vi "Quit With Parameter Code.vi"   [LabVIEW 2024, in "Integration Tests.lvlib"]
uses:
  Integration Tests.lvlib
  CLI Class/CLI.lvclass
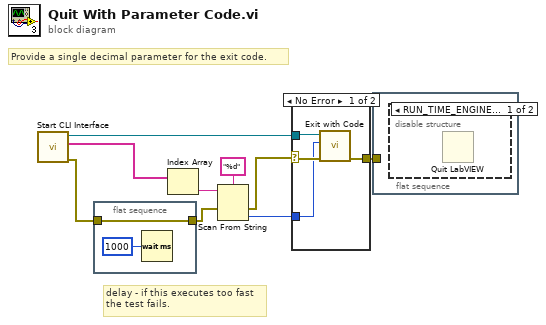
[diagram p0: block diagram]
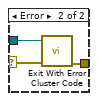
[diagram p2: hidden frame]
diagram:
  # "delay - if this executes too fast\nthe test fails."
  # "Provide a single decimal parameter for the exit code."
  n1 = call "Start CLI Interface.vi"() -> ("error out"=w2:errorcluster, "Custom Parameters"=w7:string[], "CLI out"=w9:refnum<class "CLI.lvclass">)  [unwired: 8 in, 1 out]
  n2 = flat-sequence {
    tunnel: w2 -> [w10]
    tunnel: [w10] -> w1
    frame #0 {
      n3 = Wait (ms)(milliseconds to wait=u32 1000) -> ()  [unwired: 1 out]
    }
  }
  n4 = Index Array(array=w7) -> (element=w6:string)  [unwired: 1 in]
  n5 = Scan From String(format string="%d", input string=w6, error in=w1) -> (error out=w4:errorcluster, output 1=w3:i32)  [unwired: 2 in, 2 out]
  n6 = case shown="No Error" w4 {
    selector: w4 -> [w14 w16]
    tunnel: w9 -> [w13 w18]
    tunnel: [w15 w17] -> w8
    tunnel: w3 -> [w12 _]
    frame No Error {
      n7 = call "Exit with Code.vi"("error in (no error)"=w14, "Exit Code (0)"=w12, "CLI in"=w13) -> ("error out"=w15:errorcluster)  [unwired: 8 in]
    }
    frame Error {
      n8 = call "Exit With Error Cluster Code.vi"("error in (no error)"=w16, "CLI in"=w18) -> ("error out"=w17:errorcluster)  [unwired: 9 in]
    }
  }
  n9 = flat-sequence {
    tunnel: w8 -> [_]
    frame #0 {
      n10 = disable-structure shown="RUN_TIME_ENGINE==True" {
        frame condition #0 {
          n11 = Quit LabVIEW() -> ()  [unwired: 1 in]
        }
        frame condition #1 (active) {
        }
      }
    }
  }
